vi "test_accesos_asic.vi"() -> ()   [LabVIEW 2019]
panel:
  out "Errores":i32
  out "Valor escrito.":u16 format="%.0x"
  out "Iteraciones":i32
  out "Valor Leido":u16 format="%x"
  in  "stop":bool
  out "FT_Handle":u32
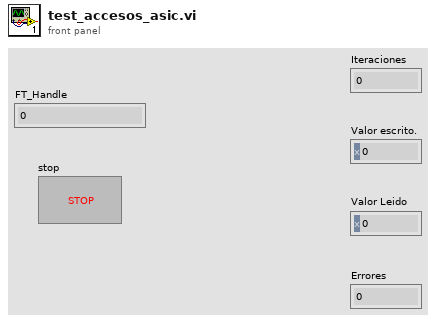
[diagram p1: front panel]
types:
  T1 = cluster{"Device Index":u32, "FT_FLAGS_OPENED":bool, "FT_FLAGS_HISPEED":bool, "Type":u32, "VID":u32, "PID":u32, "LocID":i32, "Serial Number":string, "Description":string, "FT_Handle":u32}
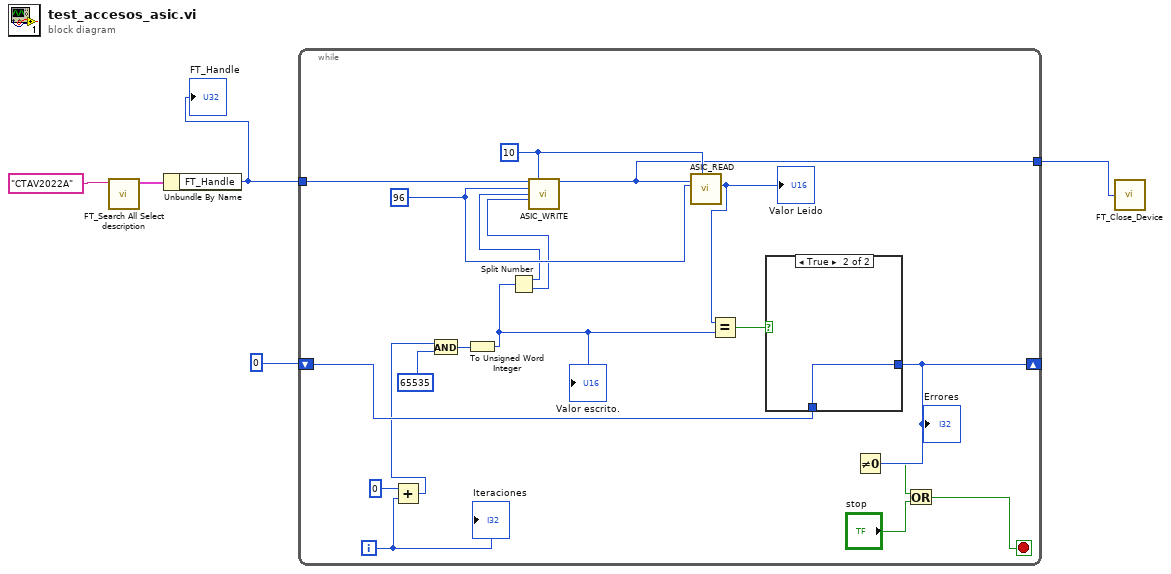
[diagram p0: block diagram]
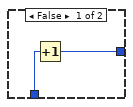
[diagram p2: hidden frame]
diagram:
  n1 = call "FT_Search All Select description.vi"("CTA Test#"="CTAV2022A") -> ("Select Ft"=w5:T1)  [unwired: 8 in, 2 out]
  n2 = Unbundle By Name(w5) -> ("FT_Handle"=w3:u32)
  "FT_Handle" <- w3
  n3 = while {
    tunnel: w3 -> [w24]
    shift-right: [w9] -> _
    shift-left: 0 -> [w18]
    tunnel: [w17] -> w2
    i -> [w12]
    stop <- w6 stop-if-true
    w22 = u8 96 ("Direccion Registro Asic")
    w23 = u32 10 ("Espera acceso USB")
    n4 = Add(x=0, y=w12) -> (x+y=w10:i32)
    n5 = And(x=w10, y=65535) -> (x .and. y?=w14:i32)
    n6 = To Unsigned Word Integer(number=w14) -> (unsigned 16bit integer=w13:u16)
    "Valor escrito." <- w13
    n7 = Split Number(x=w13) -> (hi(x)=w16:u8, lo(x)=w15:u8)
    n8 = call "ASIC_WRITE.vi"("ftHandle_in"=w24, "Espera acceso USB"=w23, "Direccion Registro Asic"=w22, "Byte Alto"=w16, "Byte Bajo"=w15) -> ("ftHandle_out"=w17:u32)  [unwired: 9 in, 1 out]
    n9 = call "ASIC_READ.vi"("Espera acceso USB"=w23, "Direccion Registro Asic"=w22, "ftHandle_in"=w17) -> ("Valor Asic"=w20:u16)  [unwired: 6 in, 2 out]
    "Valor Leido" <- w20
    n10 = Equal?(x=w20, y=w13) -> (x = y?=w19:bool)
    n11 = case shown="True" w19 {
      tunnel: w18 -> [w26 w27]
      tunnel: [w25 w27] -> w9
      frame False {
        n12 = Increment(x=w26) -> (x+1=w25:i32)
      }
      frame True {
      }
    }
    "Errores" <- w9
    n13 = Not Equal To 0?(x=w9) -> (x != 0?=w8:bool)
    n14 = Or(x=w8, y="stop") -> (x .or. y?=w6:bool)
    "Iteraciones" <- w12
  }
  n15 = call "FT_Close_Device.vi"("Handle"=w2) -> ()  [unwired: 1 out]
